vi "Configure Signaling RF UL Frequency A.vi"(8 "error in (no error)":errorcluster, 9 "UL Frequency A (0Hz)":dbl format="%#.9p", 10 "Cell Name (\"Cell Name\")":string="Cell Name", 11 "VISA resource name":refnum<visa-resource-name>) -> (0 "error out":errorcluster, 3 "VISA resource name out":refnum<visa-resource-name>)   [LabVIEW 2020, in "Rohde&Schwarz CMWXP NR FR1 Measurement.lvlib"]
doc: "Sets the user-defined frequency of point A, for the uplink.\n\nAttribute:\nRSCMWXPNRFR1M_ATTR_SIGNALING_RF_UL_FREQUENCY_A\n\nRemote-control command:\n[CONFigure:]SIGNaling:NRADio:CELL:RFSettings:UL:APOint:FREQuency"
uses:
  <instrlib>/Rohde&Schwarz CMWXP NR FR1 Measurement/Rohde&Schwarz CMWXP NR FR1 Measurement.lvlib
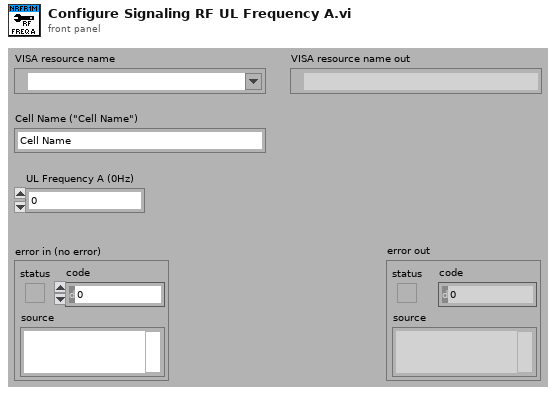
[diagram p1: front panel]
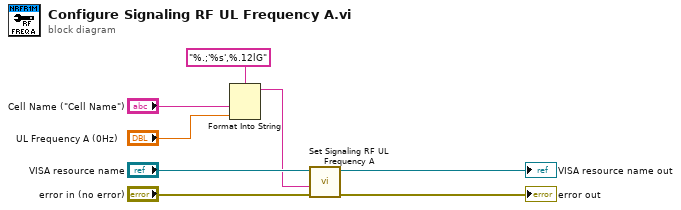
[diagram p0: block diagram]
diagram:
  n1 = Format Into String(format string="%.;'%s',%.12lG", "Cell Name (\"Cell Name\")", "UL Frequency A (0Hz)") -> (resulting string=w1:string)  [unwired: 2 in, 1 out]
  n2 = call "Set Signaling RF UL Frequency A"("error in (no error)"="error in (no error)", "Signaling RF UL Frequency A ()"=w1, "instrument handle"="VISA resource name") -> ("error out"=→"error out":errorcluster, "instrument handle out"=→"VISA resource name out":refnum<visa-resource-name>)  [unwired: 7 in]
